vi "dspMult_18x18.vi"(6 "sclr":bool, 8 "b":fxp<+/-,18,5>, 11 "a":fxp<+/-,18,5>) -> (1 "p":fxp<+/-,36,10>)   [LabVIEW 2017]
doc: "18x18 multiplier.\nUses 1 dsp block\nHas two cycles of latency.\n5 integer bits on both inputs, 10 integer bits on output"
uses:
  <vilib>/rvi/IPIntegrationNode/IPINode_Typedef/niFpgaIPINodeSupportedFamilies.ctl
  <vilib>/rvi/IPIntegrationNode/IPINode_Utilities/niFpgaIPINodeSimCore.vi
  <vilib>/rvi/XilinxIP/XIPIN_XNode/niFpgaXIPIN.xnode
  dspMult_18x18/Multiplier/Multiplier_0A309ADD3D1E4C569775C4E497293CD9.dll
  <vilib>/rvi/IPIntegrationNode/IPINode_Xnode/niFpgaIPINode.xnode
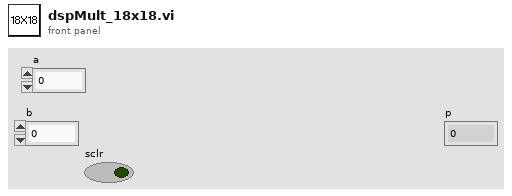
[diagram p1: front panel]
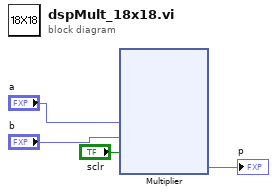
[diagram p0: block diagram]
diagram:
  n1 = xnode ("Multiplier")("a"="a", "b"="b", "sclr"="sclr") -> ("p"=→"p":fxp<+/-,36,10>)  [unwired: 1 in]
